vi "SecondSemesterExamProgramMarcoGonzalez.vi"() -> ()   [LabVIEW 2012]
doc: "This VI allows the user to choose a VI state. The user will progress through the program by deciding a state they wish to go to."
panel:
  in  "OK Button 2":bool
  in  "OK Button":bool
  out "Sum":dbl
  out "Query":string
  in  "Z":dbl
  in  "Y":dbl
  out "Option 2":string
  out "Option 1":string
  out "X":bool
  out "State":string
  # "Marco Gonzalez\nEA 3 - 6th Period\n05 / 24 / 2017"
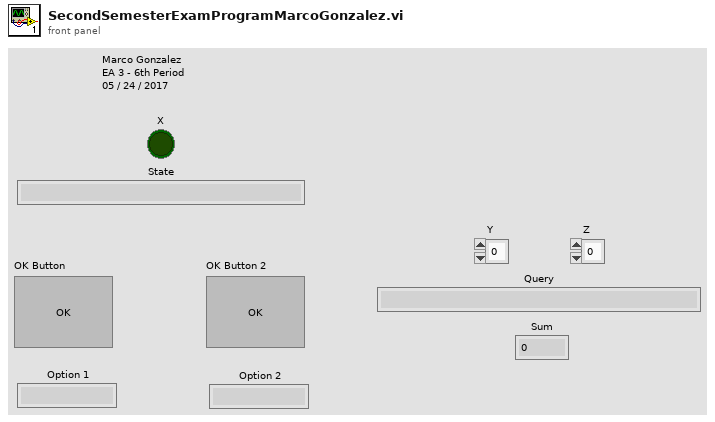
[diagram p1: front panel]
types:
  T1 = enum16{"State 1", "State 2", "State 3", "State 4"}
  T2 = enum16{"Welcome", "State 1", "State 2", "State 3", "State 4"}
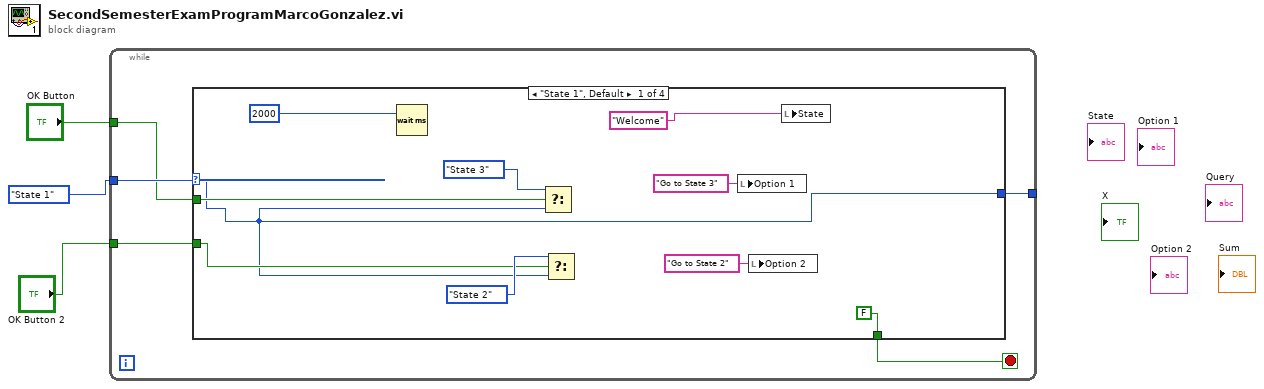
[diagram p0: block diagram]
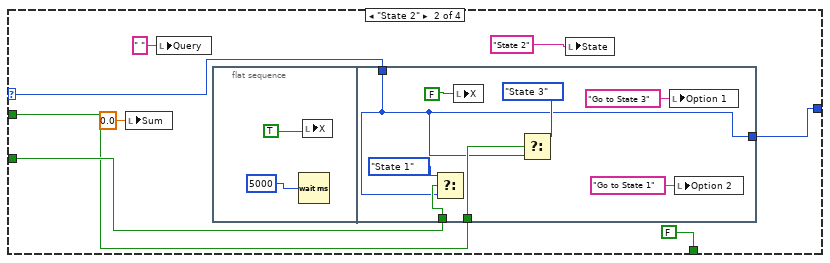
[diagram p2: hidden frame]
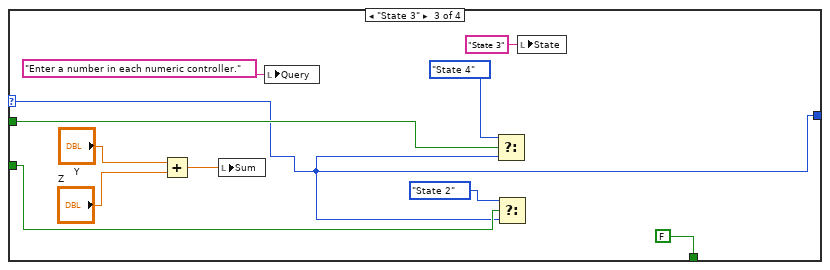
[diagram p3: hidden frame]
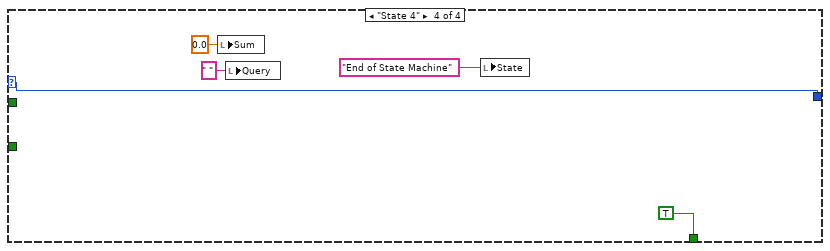
[diagram p4: hidden frame]
diagram:
  n1 = while {
    tunnel: T1."State 1" -> [w8]
    tunnel: [w7] -> _
    tunnel: "OK Button" -> [w5]
    tunnel: "OK Button 2" -> [w4]
    stop <- w6 stop-if-true
    n2 = case shown="\"State 1\", Default" w8 {
      selector: w8 -> [w9 w24 w37 w51]
      tunnel: [w9 w23 w37 w51] -> w7
      tunnel: [FALSE FALSE FALSE TRUE] -> w6
      tunnel: w4 -> [w10 w20 w38 _]
      tunnel: w5 -> [w12 w19 w40 _]
      frame "State 1", Default {
        n3 = Wait (ms)(milliseconds to wait=2000) -> ()  [unwired: 1 out]
        n4 = Select(t=T2."State 3", s=w12, f=w9) -> ()  [unwired: 1 out]
        n5 = Select(t=T2."State 2", s=w10, f=w9) -> ()  [unwired: 1 out]
        n6 = local write "Option 1"("Go to State 3" ("Option 1")) -> ()
        n7 = local write "Option 2"("Go to State 2" ("Option 2")) -> ()
        n8 = local write "State"("Welcome") -> ()
      }
      frame "State 2" {
        n9 = local write "Sum"(0.0 ("Sum")) -> ()
        n10 = local write "Query"(" " ("Query")) -> ()
        n11 = flat-sequence {
          tunnel: w24 -> [w29]
          tunnel: [w29] -> w23
          tunnel: w20 -> [w30]
          tunnel: w19 -> [w32]
          frame #0 {
            n12 = Wait (ms)(milliseconds to wait=5000) -> ()  [unwired: 1 out]
            n13 = local write "X"(TRUE) -> ()
          }
          frame #1 {
            n14 = Select(t=T1."State 1", s=w30, f=w29) -> ()  [unwired: 1 out]
            n15 = local write "X"(FALSE) -> ()
            n16 = Select(t=T1."State 3", s=w32, f=w29) -> ()  [unwired: 1 out]
            n17 = local write "Option 1"("Go to State 3" ("Option 1")) -> ()
            n18 = local write "Option 2"("Go to State 1" ("Option 2")) -> ()
          }
        }
        n19 = local write "State"("State 2") -> ()
      }
      frame "State 3" {
        n20 = Add(x="Y", y="Z") -> (x+y=w41:dbl)
        n21 = local write "Sum"(w41) -> ()
        n22 = local write "Query"("Enter a number in each numeric controller." ("Query")) -> ()
        n23 = Select(t=T1."State 4", s=w40, f=w37) -> ()  [unwired: 1 out]
        n24 = Select(t=T1."State 2", s=w38, f=w37) -> ()  [unwired: 1 out]
        n25 = local write "State"("State 3" ("State")) -> ()
      }
      frame "State 4" {
        n26 = local write "Sum"(0.0 ("Sum")) -> ()
        n27 = local write "Query"(" " ("Query")) -> ()
        n28 = local write "State"("End of State Machine" ("State")) -> ()
      }
    }
  }
